vi "Test.vi"() -> ()   [LabVIEW 2016]
uses:
  Credentials/Credentials.lvclass
  Policies/Policies.lvclass
  Session/Session.lvclass/Session.ctl
  Session/Read Active.vi
  Session/Read User.vi
  Authentication/LDAP Authentication/LDAP Authentication.lvclass
  C:/Users/robsmith/Desktop/RBAC/Authentication/Authentication.lvclass
  Session/Session.lvclass
panel:
  in  "Do Supervisor Thing":bool
  out "Greeting":string
  in  "Log In":bool
  in  "Do Admin Thing":bool
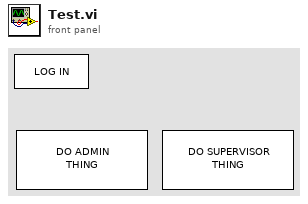
[diagram p1: front panel]
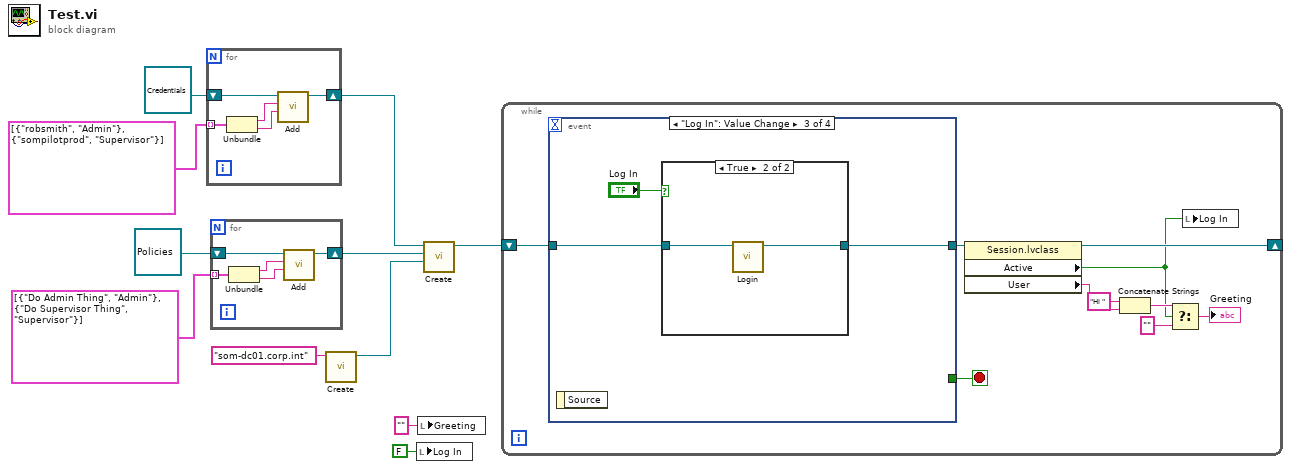
[diagram p0: block diagram]
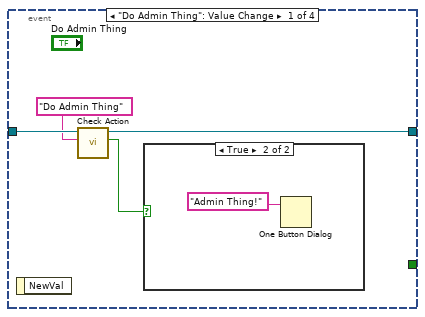
[diagram p2: hidden frame]
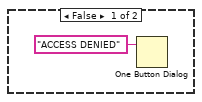
[diagram p3: hidden frame]
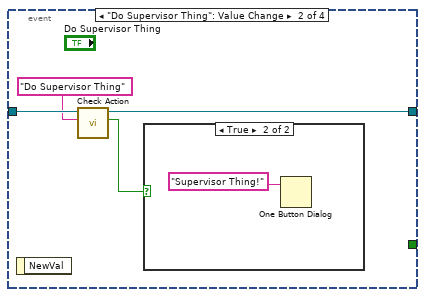
[diagram p4: hidden frame]
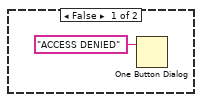
[diagram p5: hidden frame]
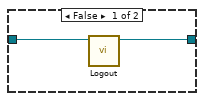
[diagram p6: hidden frame]
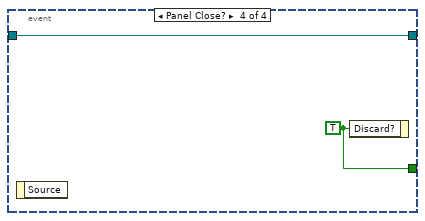
[diagram p7: hidden frame]
diagram:
  n1 = for {
    shift-right: [w16] -> w10
    shift-left: refnum<class "Credentials.lvclass"> refnum ("Credentials.lvclass") -> [w15]
    tunnel: cluster{string, string}[] [{"robsmith", "Admin"}, {"sompilotprod", "Supervisor"}] -> [w14] mode=indexing
    n2 = Unbundle(w14) -> (w13:string, w12:string)
    n3 = call "Add.vi"("Role"=w12, "User"=w13, "Credentials in"=w15) -> ("Credentials out"=w16:refnum<class "Credentials.lvclass">)  [unwired: 7 in, 1 out]
  }
  n4 = for {
    shift-right: [w20] -> w4
    shift-left: refnum<class "Policies.lvclass"> refnum ("Policies.lvclass") -> [w21]
    tunnel: cluster{string, string}[] [{"Do Admin Thing", "Admin"}, {"Do Supervisor Thing", "Supervisor"}] -> [w19] mode=indexing
    n5 = Unbundle(w19) -> (w18:string, w17:string)
    n6 = call "Add.vi"("Role"=w17, "Action"=w18, "Policies in"=w21) -> ("Policies out"=w20:refnum<class "Policies.lvclass">)  [unwired: 7 in, 1 out]
  }
  n7 = call "Create.vi"("Server"="som-dc01.corp.int") -> ("LDAP Authentication out"=w7:refnum<class "LDAP Authentication.lvclass">)  [unwired: 9 in, 1 out]
  n8 = local write "Log In"(FALSE ("Log In")) -> ()
  n9 = local write "Greeting"("" ("Greeting")) -> ()
  n10 = call "Create.vi"("Authentication"=w7, "Policies"=w4, "Credentials"=w10) -> ("Session out"=w9:refnum<class "Session.lvclass">)  [unwired: 7 in, 1 out]
  n11 = while {
    shift-right: [w28] -> _
    shift-left: w9 -> [w31]
    stop <- w29 stop-if-true
    n12 = event shown="[2] \"Log In\": Value Change" {
      selector: _ -> [_ _ _ _]
      dyn-events: _ -> [_ _ _ _]
      timeout: _ -> [_ _ _ _]
      tunnel: w31 -> [w35 w41 w46 w51]
      tunnel: [w33 w39 w45 w51] -> w30
      tunnel: [_ _ _ w52] -> w29
      event "Do Admin Thing": Value Change {
        n13 = event-data() -> ()  [unwired: 1 in, 1 out]
        n14 = call "Check Action.vi"("Action"="Do Admin Thing", "Session in"=w35) -> ("Allowed?"=w32:bool, "Session out"=w33:refnum<class "Session.lvclass">)  [unwired: 7 in, 1 out]
        n15 = case shown="True" w32 {
          frame False {
            n16 = One Button Dialog(message="ACCESS DENIED") -> ()  [unwired: 1 in, 1 out]
          }
          frame True {
            n17 = One Button Dialog(message="Admin Thing!") -> ()  [unwired: 1 in, 1 out]
          }
        }
      }
      event "Do Supervisor Thing": Value Change {
        n18 = event-data() -> ()  [unwired: 1 in, 1 out]
        n19 = call "Check Action.vi"("Action"="Do Supervisor Thing", "Session in"=w41) -> ("Allowed?"=w38:bool, "Session out"=w39:refnum<class "Session.lvclass">)  [unwired: 7 in, 1 out]
        n20 = case shown="True" w38 {
          frame False {
            n21 = One Button Dialog(message="ACCESS DENIED") -> ()  [unwired: 1 in, 1 out]
          }
          frame True {
            n22 = One Button Dialog(message="Supervisor Thing!") -> ()  [unwired: 1 in, 1 out]
          }
        }
      }
      event "Log In": Value Change {
        n23 = event-data() -> ()  [unwired: 1 in, 1 out]
        n24 = case shown="True" "Log In" {
          tunnel: w46 -> [w48 w50]
          tunnel: [w47 w49] -> w45
          frame False {
            n25 = call "Logout.vi"("Session in"=w48) -> ("Session out"=w47:refnum<class "Session.lvclass">)  [unwired: 9 in, 1 out]
          }
          frame True {
            n26 = call "Login.vi"("Session in"=w50) -> ("Session out"=w49:refnum<class "Session.lvclass">)  [unwired: 9 in, 1 out]
          }
        }
      }
      event Panel Close? {
        w52 = TRUE ("Discard?")
        n27 = event-data() -> ()  [unwired: 1 in, 1 out]
        n28 = event-data("Discard?"=w52) -> ()  [unwired: 1 in, 1 out]
      }
    }
    n29 = property class="Session.lvclass"(reference=w30) -> (reference out=w28:refnum<class "Session.lvclass">, "Active"=w22:bool, "User"=w27:string)  [unwired: 1 in, 1 out]
    n30 = Concatenate Strings("Hi " ("string"), w27) -> (w25:string)
    n31 = Select(t=w25, s=w22, f="") -> (s? t:f=→"Greeting":string)
    n32 = local write "Log In"(w22) -> ()
  }
